vi "Brent with Derivatives Prep (VI).vi"(4 "sign":i32(ring) items=["y=f(x)", "y=-f(x)"], 5 "accuracy":dbl format="%.2f", 6 "data":variant, 7 "f(x)":T1, 8 "error in":i32, 9 "values":T2 {"c (start)" format="%.2f"; "b (start)" format="%.2f"; "a (start)" format="%.2f"}, 10 "inner case":bool, 11 "outer case":bool) -> (0 "error out":i32, 2 "f(minimum)":dbl format="%.2f", 3 "minimum":dbl format="%.2f")   [LabVIEW 2014, in "NI_Gmath.lvlib"]
uses:
  NI_Gmath.lvlib
  functionRefnum.ctl
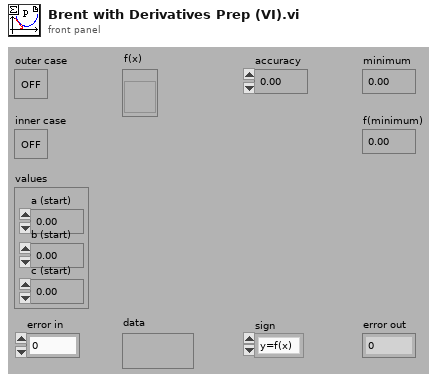
[diagram p1: front panel]
types:
  T1 = typedef "NI_Gmath.lvlib/functionRefnum.ctl" = refnum<vi>
  T2 = cluster{"a (start)":dbl, "b (start) ":dbl, "c (start)":dbl}
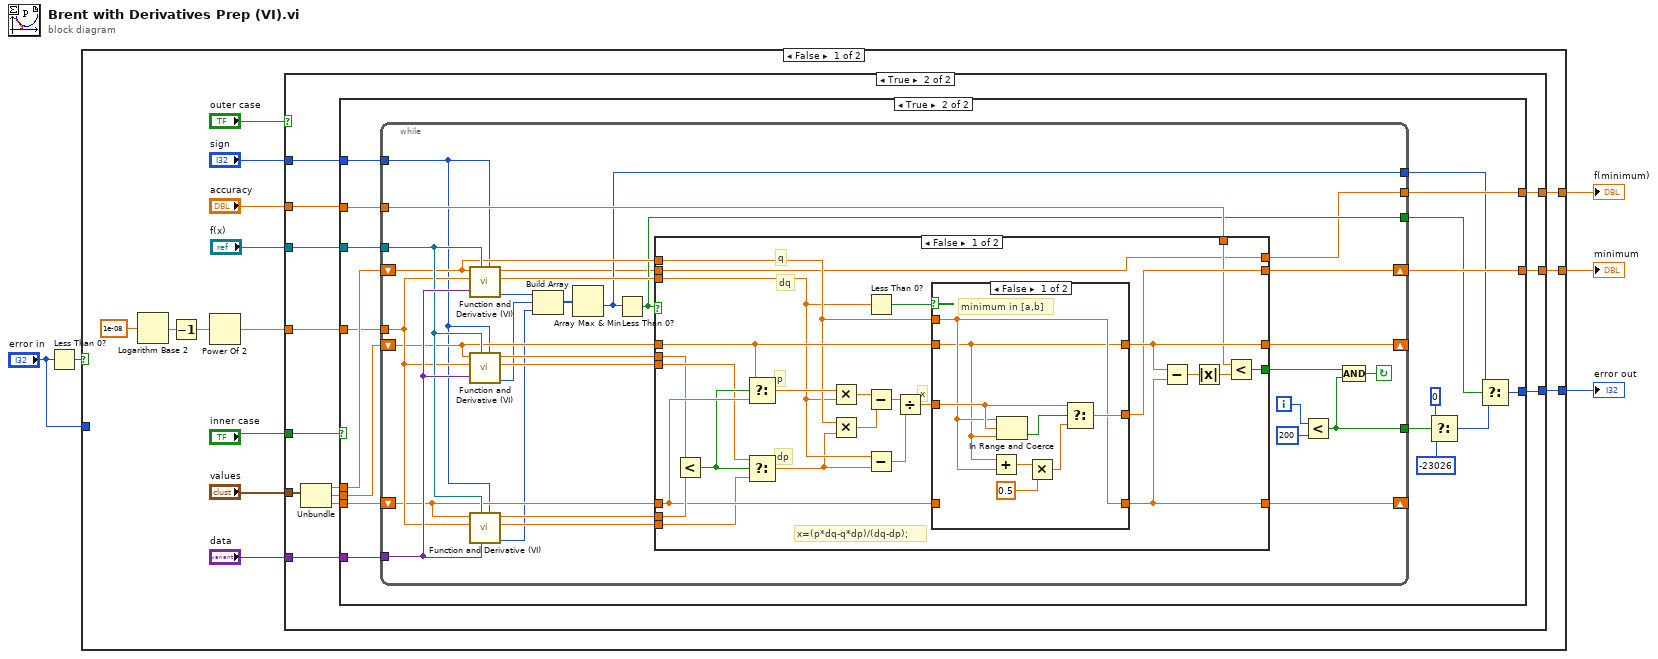
[diagram p0: block diagram]
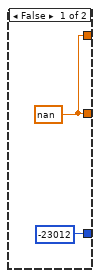
[diagram p2: hidden frame]
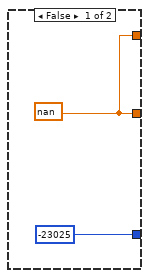
[diagram p3: hidden frame]
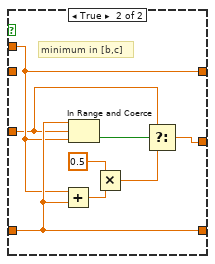
[diagram p4: hidden frame]
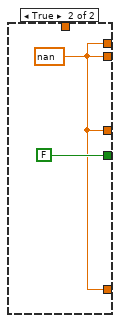
[diagram p5: hidden frame]
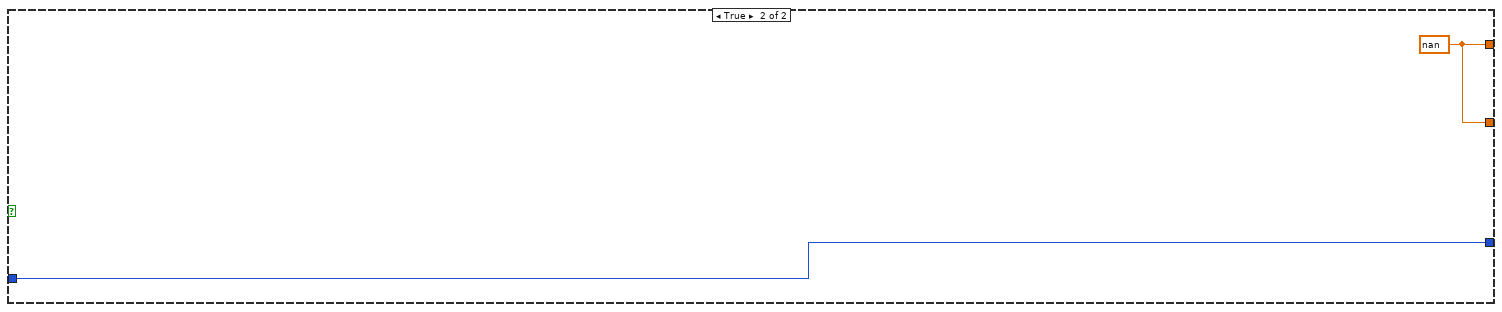
[diagram p6: hidden frame]
diagram:
  n1 = Less Than 0?(x="error in") -> (x < 0?=w2:bool)
  n2 = case shown="False" w2 {
    tunnel: [w18 w126] -> w3
    tunnel: [w15 w127] -> w5
    tunnel: [w14 w127] -> w4
    tunnel: "error in" -> [_ w126]
    frame False {
      n3 = Logarithm Base 2(1:1e-08) -> (0:w11:dbl)
      n4 = Decrement(x=w11) -> (x-1=w10:dbl)
      n5 = Power Of 2(x=w10) -> (2^x=w9:dbl)
      n6 = case shown="True" "outer case" {
        tunnel: [w21 w34] -> w15
        tunnel: [w21 w33] -> w14
        tunnel: "inner case" -> [_ w32]
        tunnel: "accuracy" -> [_ w31]
        tunnel: [-23012 w30] -> w18
        tunnel: "values" -> [_ w29]
        tunnel: w9 -> [_ w25]
        tunnel: "f(x)" -> [_ w24]
        tunnel: "data" -> [_ w23]
        tunnel: "sign" -> [_ w22]
        frame False {
          w21 = nan
        }
        frame True {
          n7 = Unbundle(w29) -> ("a (start)"=w28:dbl, "b (start)"=w27:dbl, "c (start)"=w26:dbl)
          n8 = case shown="True" w32 {
            tunnel: w27 -> [_ w53]
            tunnel: w28 -> [_ w52]
            tunnel: w26 -> [_ w51]
            tunnel: [w36 w50] -> w33
            tunnel: [w36 w49] -> w34
            tunnel: w31 -> [_ w48]
            tunnel: [-23025 w39] -> w30
            tunnel: w25 -> [_ w47]
            tunnel: w24 -> [_ w46]
            tunnel: w23 -> [_ w45]
            tunnel: w22 -> [_ w38]
            frame False {
              w36 = nan
            }
            frame True {
              n9 = while {
                tunnel: [w74] -> w44
                tunnel: w48 -> [w77]
                tunnel: [w54] -> w49
                tunnel: w47 -> [w70]
                shift-left: w51 -> [w68]
                shift-right: [w80] -> _
                shift-left: w52 -> [w65]
                shift-right: [w78] -> w50
                shift-left: w53 -> [w69]
                shift-right: [w81] -> _
                tunnel: w46 -> [w71]
                tunnel: w45 -> [w82]
                tunnel: [w58] -> w41
                tunnel: w38 -> [w57]
                tunnel: [w56] -> w37
                i -> [w76]
                stop <- w72 continue-if-true
                n10 = call "Function and Derivative (VI).vi"("sign"=w57, "data"=w82, "f(x)"=w71, "(x+h)-x"=w70, "x"=w65) -> ("error"=w62:i32, "df(x)/dx"=w63:dbl, "f(x)"=w55:dbl)  [unwired: 4 out]
                n11 = call "Function and Derivative (VI).vi"("sign"=w57, "data"=w82, "f(x)"=w71, "(x+h)-x"=w70, "x"=w69) -> ("error"=w61:i32, "df(x)/dx"=w67:dbl, "f(x)"=w64:dbl)  [unwired: 4 out]
                n12 = call "Function and Derivative (VI).vi"("sign"=w57, "data"=w82, "f(x)"=w71, "(x+h)-x"=w70, "x"=w68) -> ("error"=w60:i32, "df(x)/dx"=w66:dbl, "f(x)"=w79:dbl)  [unwired: 4 out]
                n13 = Build Array(w62, w61, w60) -> (w59:i32[])
                n14 = Array Max & Min(array=w59) -> (min value=w58:i32)  [unwired: 3 out]
                n15 = Less Than 0?(x=w58) -> (x < 0?=w56:bool)
                n16 = case shown="False" w56 {
                  tunnel: [w106 w124] -> w81
                  tunnel: [w105 w124] -> w80
                  tunnel: w79 -> [w102 _]
                  tunnel: [w101 w124] -> w78
                  tunnel: w77 -> [w100 _]
                  tunnel: [w99 FALSE] -> w73
                  tunnel: w69 -> [w98 _]
                  tunnel: w68 -> [w97 _]
                  tunnel: w67 -> [w95 _]
                  tunnel: w66 -> [w94 _]
                  tunnel: w65 -> [w87 _]
                  tunnel: w64 -> [w86 _]
                  tunnel: w63 -> [w85 _]
                  tunnel: w55 -> [w83 _]
                  tunnel: [w83 w124] -> w54
                  frame False {
                    # "x=(p*dq-q*dp)/(dq-dp);"
                    # "x"
                    # "dq"
                    # "q"
                    # "dp"
                    # "p"
                    n17 = Less?(x=w86, y=w102) -> (x < y?=w96:bool)
                    n18 = Select(t=w98, s=w96, f=w97) -> (s? t:f=w93:dbl)
                    n19 = Select(t=w95, s=w96, f=w94) -> (s? t:f=w84:dbl)
                    n20 = Multiply(x=w93, y=w85) -> (x*y=w92:dbl)
                    n21 = Multiply(x=w87, y=w84) -> (x*y=w91:dbl)
                    n22 = Less Than 0?(x=w85) -> (x < 0?=w107:bool)
                    n23 = Subtract(x=w92, y=w91) -> (x-y=w90:dbl)
                    n24 = Subtract(x=w85, y=w84) -> (x-y=w89:dbl)
                    n25 = Divide(x=w90, y=w89) -> (x/y=w88:dbl)
                    n26 = case shown="False" w107 {
                      tunnel: w88 -> [w112 w118]
                      tunnel: w87 -> [w109 w122]
                      tunnel: w97 -> [_ w123]
                      tunnel: w98 -> [w108 _]
                      tunnel: [w108 w122] -> w106
                      tunnel: [w110 w116] -> w101
                      tunnel: [w109 w123] -> w105
                      frame False {
                        # "minimum in [a,b]"
                        n27 = Add(x=w108, y=w109) -> (x+y=w115:dbl)
                        n28 = In Range and Coerce(upper limit=w109, x=w112, lower limit=w108) -> (In Range?=w113:bool)  [unwired: 1 out]
                        n29 = Multiply(x=w115, y=0.5) -> (x*y=w111:dbl)
                        n30 = Select(t=w112, s=w113, f=w111) -> (s? t:f=w110:dbl)
                      }
                      frame True {
                        # "minimum in [b,c]"
                        n31 = Add(x=w122, y=w123) -> (x+y=w121:dbl)
                        n32 = In Range and Coerce(upper limit=w123, x=w118, lower limit=w122) -> (In Range?=w119:bool)  [unwired: 1 out]
                        n33 = Multiply(x=0.5, y=w121) -> (x*y=w117:dbl)
                        n34 = Select(t=w118, s=w119, f=w117) -> (s? t:f=w116:dbl)
                      }
                    }
                    n35 = Subtract(x=w106, y=w105) -> (x-y=w104:dbl)
                    n36 = Absolute Value(x=w104) -> (abs(x)=w103:dbl)
                    n37 = Less?(x=w100, y=w103) -> (x < y?=w99:bool)
                  }
                  frame True {
                    w124 = nan
                  }
                }
                n38 = Less?(x=w76, y=200) -> (x < y?=w74:bool)
                n39 = Compound Arithmetic op=AND(w73, w74) -> (w72:bool)
              }
              n40 = Select(t=0, s=w44, f=-23026) -> (s? t:f=w40:i32)
              n41 = Select(t=w41, s=w37, f=w40) -> (s? t:f=w39:i32)
            }
          }
        }
      }
    }
    frame True {
      w127 = nan
    }
  }
  "f(minimum)" <- w5
  "minimum" <- w4
  "error out" <- w3
